vi "svl_Clip to Baseline.vi"(1 "baseline":dbl format="%.2f", 2 "waterfall data":dbl[][](array[numeric]) format="%.2f") -> (0 "clipped data":dbl[][](array[numeric]) format="%.2f")   [LabVIEW 2017]
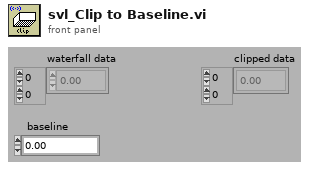
[diagram p1: front panel]
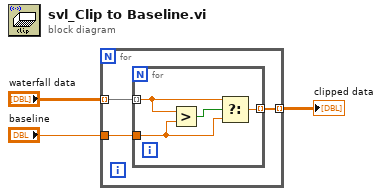
[diagram p0: block diagram]
diagram:
  n1 = for {
    tunnel: "waterfall data" -> [w4] mode=indexing
    tunnel: "baseline" -> [w6]
    tunnel: [w5] -> w3 mode=indexing
    n2 = for {
      tunnel: w4 -> [w7] mode=indexing
      tunnel: w6 -> [w9]
      tunnel: [w8] -> w5 mode=indexing
      n3 = Greater?(x=w7, y=w9) -> (0:w10:bool)
      n4 = Select(t=w7, s=w10, f=w9) -> (s? t:f=w8:dbl)
    }
  }
  "clipped data" <- w3
